vi "convertEntryParaTableToArray.vi"(8 "error in":errorcluster, 11 "entryParaTbl":string[][](array[string])) -> (0 "error out":errorcluster, 3 "contArr":string[](array[string]))   [LabVIEW 2010]
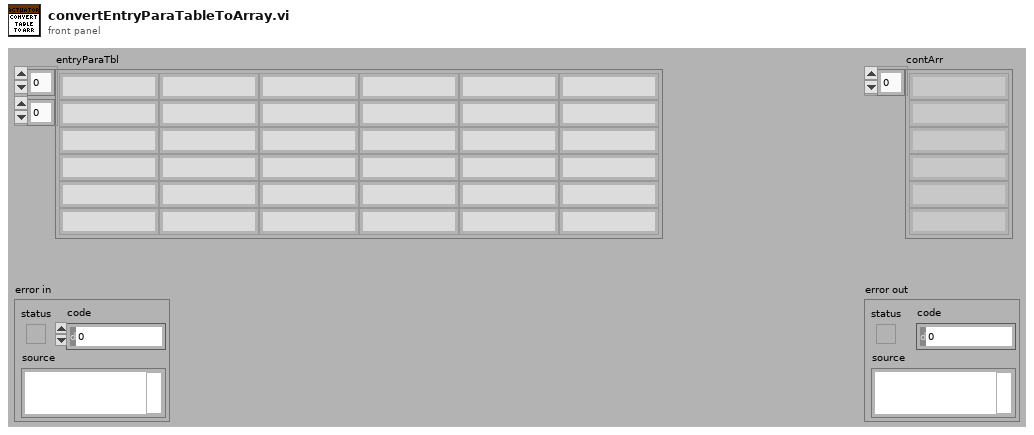
[diagram p1: front panel]
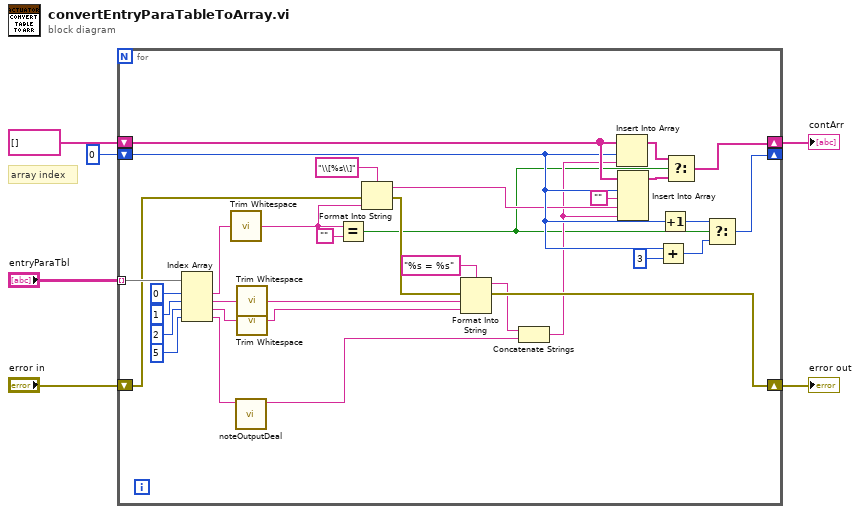
[diagram p0: block diagram]
diagram:
  # "array index"
  n1 = for {
    tunnel: "entryParaTbl" -> [w38] mode=indexing
    shift-right: [w26] -> w2
    shift-left: string[] [] ("Value") -> [w28]
    shift-right: [w23] -> w1
    shift-left: "error in" -> [w24]
    shift-right: [w25] -> _
    shift-left: 0 ("input 1") -> [w27]
    n2 = Index Array(array=w38, index #1=0 ("index"), index #2=1 ("index"), index #3=2 ("index"), index #4=5 ("index")) -> (element #1=w33:string, element #2=w34:string, element #3=w32:string, element #4=w30:string)
    n3 = call <vilib>:"Trim Whitespace.vi"("string"=w33) -> ("trimmed string"=w31:string)  [unwired: 1 in]
    n4 = call "noteOutputDeal.vi"("note in editor"=w30) -> ("note output"=w29:string)  [unwired: 10 in]
    n5 = call <vilib>:"Trim Whitespace.vi"("string"=w34) -> ("trimmed string"=w8:string)  [unwired: 1 in]
    n6 = call <vilib>:"Trim Whitespace.vi"("string"=w32) -> ("trimmed string"=w7:string)  [unwired: 1 in]
    n7 = Equal?(x=w31, y="") -> (x = y?=w12:bool)
    n8 = Format Into String(format string="\\[%s\\]", error in=w24, w31) -> (resulting string=w15:string, error out=w17:errorcluster)  [unwired: 1 in]
    n9 = Format Into String(format string="%s = %s", error in=w17, w8, w7) -> (resulting string=w20:string, error out=w23:errorcluster)  [unwired: 1 in]
    n10 = Concatenate Strings(w20, w29) -> (w14:string)
    n11 = Insert Into Array(array=w28, index=w27, new element=w14) -> (w19:string[])
    n12 = Insert Into Array(array=w28, index=w27, new element #1="", new element #2=w15, new element #3=w14) -> (w13:string[])
    n13 = Add(x=w27, y=3) -> (x+y=w10:i32)
    n14 = Increment(x=w27) -> (x+1=w11:i32)
    n15 = Select(t=w19, s=w12, f=w13) -> (s? t:f=w26:string[])
    n16 = Select(t=w11, s=w12, f=w10) -> (s? t:f=w25:i32)
  }
  "contArr" <- w2
  "error out" <- w1
